vi "AddAllAvailable.vi"(0 "objects":T1, 11 "error in":errorcluster) -> (15 "error out":errorcluster)   [LabVIEW 2017, in "JSON_RPC_Interface editor node.lvclass"]
uses:
  JSON_RPC_Interface editor node.lvclass
  <vilib>/NI/DCAF/Tag Editor Core/Table API/Table Manager/object ref.ctl
  <vilib>/NI/DCAF/Tag Editor Core/Configuration Editor/Classes/Engine Parent/Engine Parent Editor Node.lvclass
  <vilib>/NI/DCAF/Tag Editor Core/Configuration Editor/Classes/Module editor node/module editor node.lvclass
  <vilib>/NI/Module Execution Interface/Engine Configuration/engine configuration.lvclass/engine configuration.ctl
  Mappings.ctl
  module/configuration/Line.ctl
  <vilib>/NI/Tag Bus Module Framework/channel/TBM channel.lvclass
  C:/Program Files (x86)/National Instruments/LabVIEW 2017/vi.lib/NI/Tag Bus/tag/tag descriptor.lvclass
  Map.ctl
  <vilib>/NI/Tag Bus Module Framework/channel/channel classification.ctl
  <vilib>/NI/Tag Bus/tag/tag descriptor.lvclass/tag descriptor.ctl
  <vilib>/NI/Tag Bus Module Framework/channel/TBM channel.lvclass/TBM channel.ctl
  <vilib>/NI/Tag Bus/tag/read tag name.vi
  <vilib>/NI/Tag Bus/tag/read data type.vi
  <vilib>/NI/Tag Bus/tag/write tag name.vi
  <vilib>/NI/Tag Bus Module Framework/channel/Write channel classification.vi
  <vilib>/NI/Tag Bus/tag/write data type.vi
  <vilib>/NI/Tag Bus/tag/tag descriptor.lvclass
  <vilib>/NI/Module Execution Interface/Engine Configuration/engine configuration.lvclass
  module/configuration/JSON_RPC_Interface configuration.lvclass
  <vilib>/NI/DCAF/Tag Editor Core/Table API/Table Manager/Table Manager.lvclass
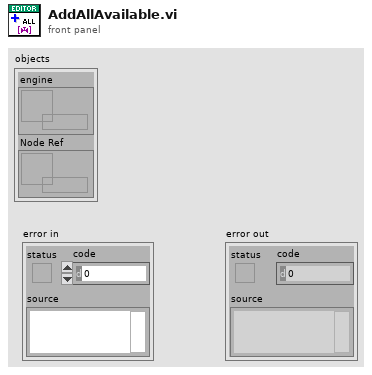
[diagram p1: front panel]
types:
  T1 = typedef "Table Manager.lvlib/Table Manager.lvclass/object ref.ctl" = cluster{"engine":refnum<data-value>, "Node Ref":refnum<data-value>}
  T2 = typedef "TBM channel.lvclass/channel classification.ctl" = enum16{"input data", "output data", "processing parameter", "processing result"}
  T3 = typedef "JSON_RPC_Interface editor node.lvclass/Map.ctl" = cluster{"channel":refnum<class "TBM channel.lvclass">, "tag name":string}
  T4 = typedef "JSON_RPC_Interface editor node.lvclass/Mappings.ctl" = cluster{"Line":T5, "Maps":T3[]}
  T5 = typedef "JSON_RPC_Interface configuration.lvclass/Line.ctl" = cluster{"channel":refnum<class "TBM channel.lvclass">}
  T6 = typedef "tag bus.lvlib/tag descriptor.lvclass/Data Type.ctl" = enum16{"Double", "Single", "I64", "I32", "I16", "I8", "U64", "U32", "U16", "U8", "Boolean", "String", "Array of Double", "Array of Single", "Array of I64", "Array of I32", "Array of I16", "Array of I8", "Array of U64", "Array of U32", "Array of U16", "Array of U8", "Array of Boolean", "Array of String"}
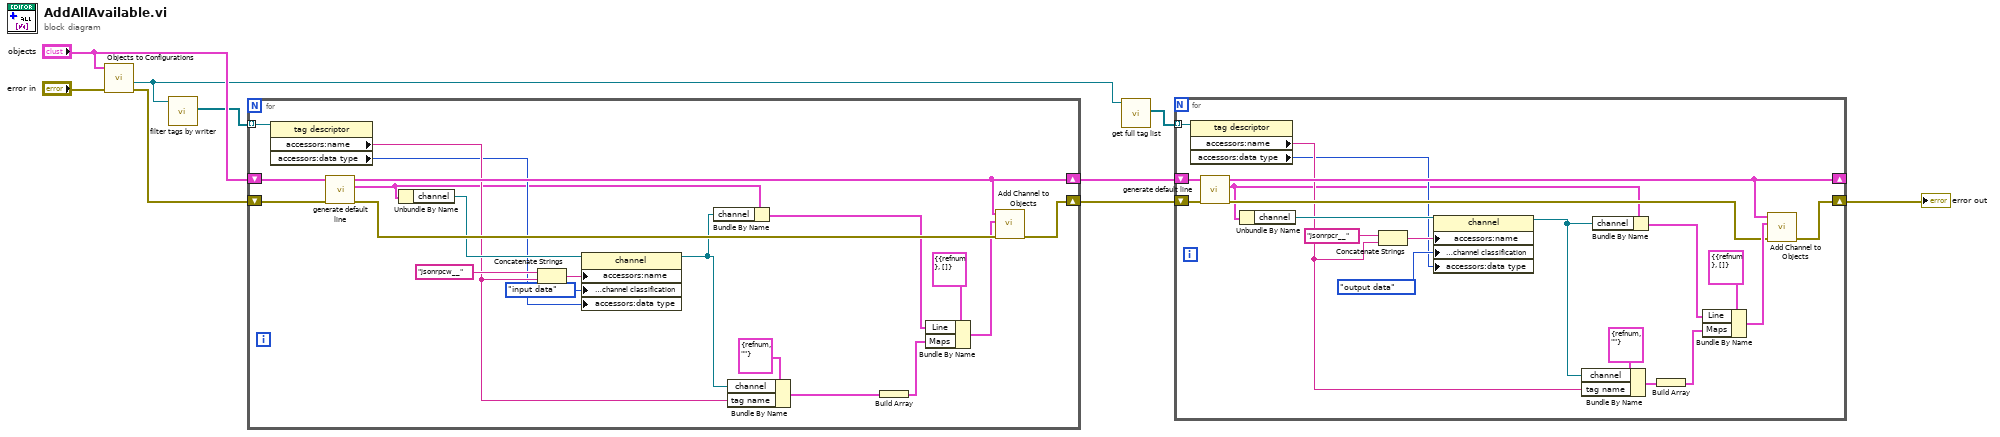
[diagram p0: block diagram]
diagram:
  n1 = call "Objects to Configurations.vi"("error in (no error)"="error in", "Objects in"="objects") -> ("error out"=w8:errorcluster, "engine configuration out"=w6:refnum<class "engine configuration.lvclass">)  [unwired: 7 in, 1 out]
  n2 = call <vilib>:"filter tags by writer.vi"("engine configuration in"=w6) -> ("tag list"=w1:refnum<class "tag descriptor.lvclass">[])  [unwired: 9 in, 1 out]
  n3 = for {
    shift-right: [w26] -> w3
    shift-left: w8 -> [w29]
    shift-right: [w24] -> w4
    shift-left: "objects" -> [w28]
    tunnel: w1 -> [w25] mode=indexing
    n4 = property class="tag descriptor"(reference=w25) -> ("accessors:name"=w15:string, "accessors:data type"=w13:T6)  [unwired: 1 in, 2 out]
    n5 = call "generate default line.vi"("error in"=w29, "objects in"=w28) -> ("error out"=w27:errorcluster, "Line"=w12:T5, "objects out"=w24:T1)  [unwired: 7 in]
    n6 = Unbundle By Name(w12) -> ("channel"=w18:refnum<class "TBM channel.lvclass">)
    n7 = Concatenate Strings("jsonrpcw__" ("string"), w15) -> (w17:string)
    n8 = property class="channel"(reference=w18, "accessors:name"=w17, "data access:channel classification"=channel_classification."input data" ("channel classification"), "accessors:data type"=w13) -> (reference out=w11:refnum<class "TBM channel.lvclass">)  [unwired: 1 in, 1 out]
    n9 = Bundle By Name(cluster=w12, "channel"=w11) -> (w10:T5)
    n10 = Bundle By Name(cluster=T3 {"channel"=refnum, "tag name"=""} ("Map"), "channel"=w11, "tag name"=w15) -> (w21:T3)
    n11 = Build Array(w21) -> (w20:T3[])
    n12 = Bundle By Name(cluster=T4 {"Line"={"channel"=refnum}, "Maps"=[]} ("Line Item in"), "Line"=w10, "Maps"=w20) -> (w19:T4)
    n13 = call "Add Channel to Objects.vi"("error in"=w27, "Line Item in"=w19, "Objects in"=w24) -> ("error out"=w26:errorcluster)  [unwired: 7 in, 1 out]
  }
  n14 = call <vilib>:"get full tag list.vi"("engine configuration in"=w6) -> ("tag list"=w5:refnum<class "tag descriptor.lvclass">[])  [unwired: 9 in, 1 out]
  n15 = for {
    tunnel: w5 -> [w46] mode=indexing
    shift-right: [w47] -> _
    shift-left: w4 -> [w49]
    shift-right: [w39] -> w2
    shift-left: w3 -> [w48]
    n16 = property class="tag descriptor"(reference=w46) -> ("accessors:name"=w35:string, "accessors:data type"=w33:T6)  [unwired: 1 in, 2 out]
    n17 = call "generate default line.vi"("error in"=w48, "objects in"=w49) -> ("error out"=w40:errorcluster, "Line"=w32:T5, "objects out"=w47:T1)  [unwired: 7 in]
    n18 = Unbundle By Name(w32) -> ("channel"=w38:refnum<class "TBM channel.lvclass">)
    n19 = Concatenate Strings("jsonrpcr__" ("string"), w35) -> (w37:string)
    n20 = property class="channel"(reference=w38, "accessors:name"=w37, "data access:channel classification"=channel_classification."output data" ("channel classification"), "accessors:data type"=w33) -> (reference out=w31:refnum<class "TBM channel.lvclass">)  [unwired: 1 in, 1 out]
    n21 = Bundle By Name(cluster=T3 {"channel"=refnum, "tag name"=""} ("Map"), "channel"=w31, "tag name"=w35) -> (w44:T3)
    n22 = Bundle By Name(cluster=w32, "channel"=w31) -> (w30:T5)
    n23 = Build Array(w44) -> (w45:T3[])
    n24 = Bundle By Name(cluster=T4 {"Line"={"channel"=refnum}, "Maps"=[]} ("Line Item in"), "Line"=w30, "Maps"=w45) -> (w41:T4)
    n25 = call "Add Channel to Objects.vi"("error in"=w40, "Line Item in"=w41, "Objects in"=w47) -> ("error out"=w39:errorcluster)  [unwired: 7 in, 1 out]
  }
  "error out" <- w2
